vi "Get TimeStamp Column Data.vi"(9 "First T0":timestamp, 10 "Array Size":i32, 11 "CSV Settings":T1) -> (3 "Timestamp Column Data":string[][](array[string]))   [LabVIEW 2022 SP3, in "CSV Export.lvlib" / "CSV Export.lvclass"]
uses:
  CSV Export.lvclass
  Controls/CSV Export Settings.ctl
  CSV Export.lvclass/CSV Export.ctl
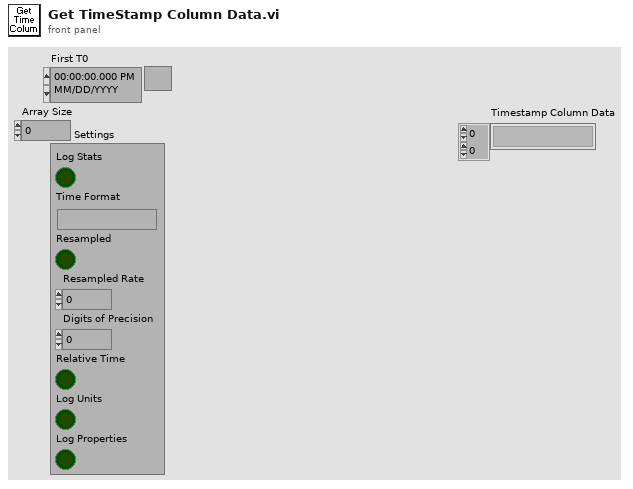
[diagram p1: front panel]
types:
  T1 = typedef "CSV Export.lvlib/CSV Export.lvclass/CSV Export Settings.ctl" = cluster{"Log Stats":bool, "Time Format":string, "Resampled":bool, "Resampled Rate":dbl, "Digits of Precision":u32, "Relative Time":bool, "Log Units":bool, "Log Properties":bool}
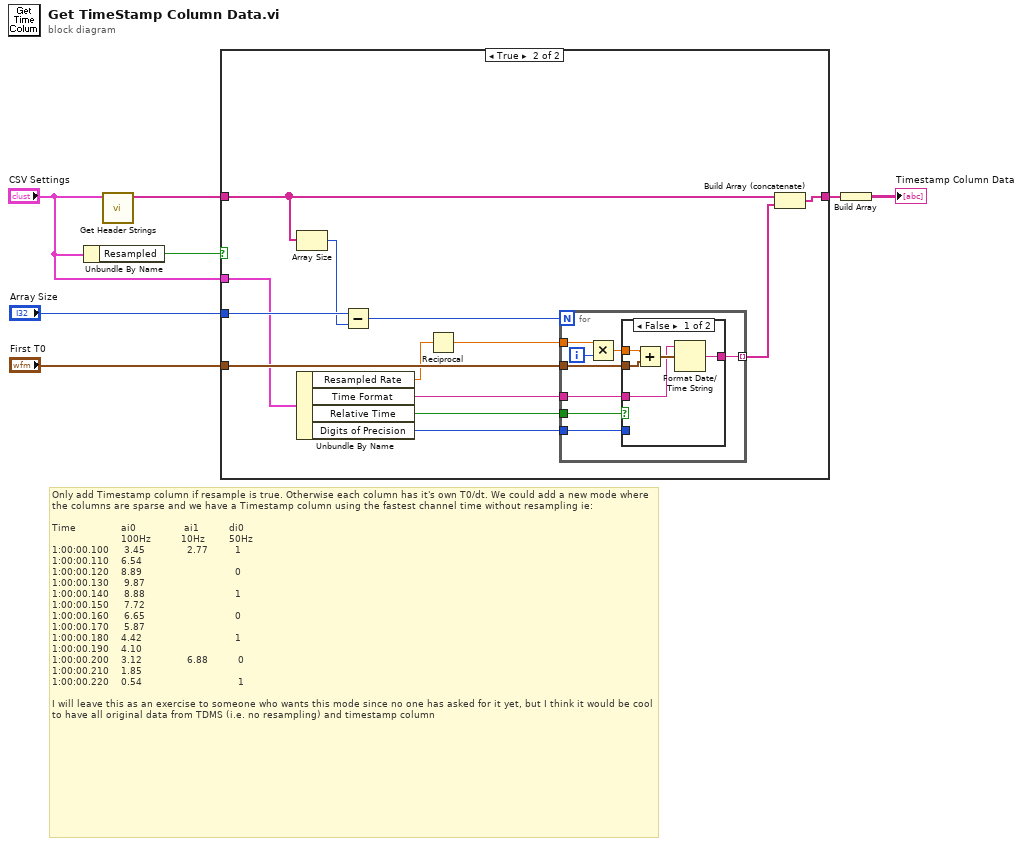
[diagram p0: block diagram]
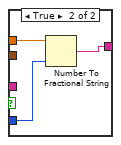
[diagram p3: hidden frame]
diagram:
  # "Only add Timestamp column if resample is true. Otherwise each column has it's own T0/dt. We could add a new mode where the columns are sparse and we have a Timestamp column using the fastest channel time without resampling ie:\n\nTime               ai0                ai1          di0\n                       100Hz          10Hz        50Hz\n1:00:00.100     3.45              2.77         1\n1:00:00.110    6.54\n1:00:00.120    8.89                               0\n1:00:00.130     9.87                                  \n1:00:00.140     8.88                              1\n1:00:00.150     7.72              \n1:00:00.160     6.65                              0\n1:00:00.170     5.87\n1:00:00.180    4.42                               1 \n1:00:00.190    4.10\n1:00:00.200    3.12               6.88          0\n1:00:00.210    1.85\n1:00:00.220    0.54                                1\n\nI will leave this as an exercise to someone who wants this mode since no one has asked for it yet, but I think it would be cool to have all original data from TDMS (i.e. no resampling) and timestamp column"
  n1 = Unbundle By Name("CSV Settings") -> ("Resampled"=w7:bool)
  n2 = call "Get Header Strings.vi"("CSV Settings"="CSV Settings") -> ("Header Values"=w3:string[])  [unwired: 10 in]
  n3 = case shown="True" w7 {
    tunnel: "Array Size" -> [_ w21]
    tunnel: "First T0" -> [_ w18]
    tunnel: [w8 w16] -> w2
    tunnel: "CSV Settings" -> [_ w10]
    tunnel: w3 -> [w8 w9]
    frame False {
    }
    frame True {
      n4 = Array Size(array=w9) -> (size(s)=w15:i32)
      n5 = Unbundle By Name(w10) -> ("Resampled Rate"=w11:dbl, "Time Format"=w12:string, "Relative Time"=w13:bool, "Digits of Precision"=w14:u32)
      n6 = Subtract(x=w21, y=w15) -> (x-y=w20:i32)
      n7 = Reciprocal(x=w11) -> (1/x=w19:dbl)
      n8 = for {
        N: w20 -> [_]
        tunnel: w19 -> [w29]
        tunnel: w18 -> [w26]
        tunnel: w12 -> [w25]
        tunnel: [w24] -> w17 mode=indexing
        tunnel: w13 -> [w23]
        tunnel: w14 -> [w22]
        i -> [w28]
        n9 = Multiply(x=w29, y=w28) -> (x*y=w27:dbl)
        n10 = case shown="False" w23 {
          tunnel: w27 -> [w34 w37]
          tunnel: w26 -> [w33 _]
          tunnel: w25 -> [w31 _]
          tunnel: [w30 w36] -> w24
          tunnel: w22 -> [_ w35]
          frame False {
            n11 = Add(x=w34, y=w33) -> (x+y=w32:timestamp)
            n12 = Format Date/Time String(time format string (%c)=w31, seconds (now)=w32) -> (date/time string=w30:string)  [unwired: 1 in]
          }
          frame True {
            n13 = Number To Fractional String(number=w37, precision (6)=w35) -> (F-format string=w36:string)  [unwired: 2 in]
          }
        }
      }
      n14 = Build Array (concatenate)(w9, w17) -> (w16:string[])
    }
  }
  n15 = Build Array(w2) -> (→"Timestamp Column Data":string[][])
